vi "subBuildSpecAndReplaceLibrary.vi"(8 "error in (no error)":errorcluster, 9 "Spec and project refs":map{string, T2}(c390), 10 "FileInfo":T1, 11 "VI in":refnum<vi>) -> (0 "error out":errorcluster, 1 "Loose files":path[](array[path]), 2 "Result":string, 3 "Message":string)   [LabVIEW 2020, in "SolutionBuilder.lvlib" / "SolutionBuilder.lvclass"]
uses:
  SolutionBuilder.lvclass
  Private/SpecAndProject.ctl
  Private/FileInfo.ctl
  <vilib>/Utility/miscctls.llb/LVReplaceWithSaveOptionEnum.ctl
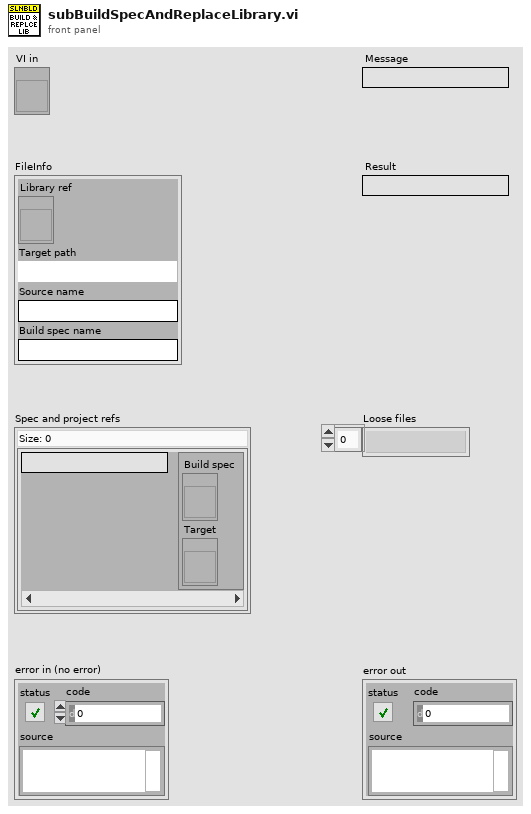
[diagram p1: front panel]
types:
  T1 = typedef "SolutionBuilder.lvlib/SolutionBuilder.lvclass/FileInfo.ctl" = cluster{"Library ref":refnum<vi>, "Target path":path, "Source name":string, "Build spec name":string}
  T2 = typedef "SolutionBuilder.lvlib/SolutionBuilder.lvclass/SpecAndProject.ctl" = cluster{"Build spec":refnum<vi>, "Target":refnum<vi>}
  T3 = typedef "LVReplaceWithSaveOptionEnum.ctl" = enum16{"Save All Without Prompts", "Save All With Prompts", "Do Not Save (Retain In Memory)"}
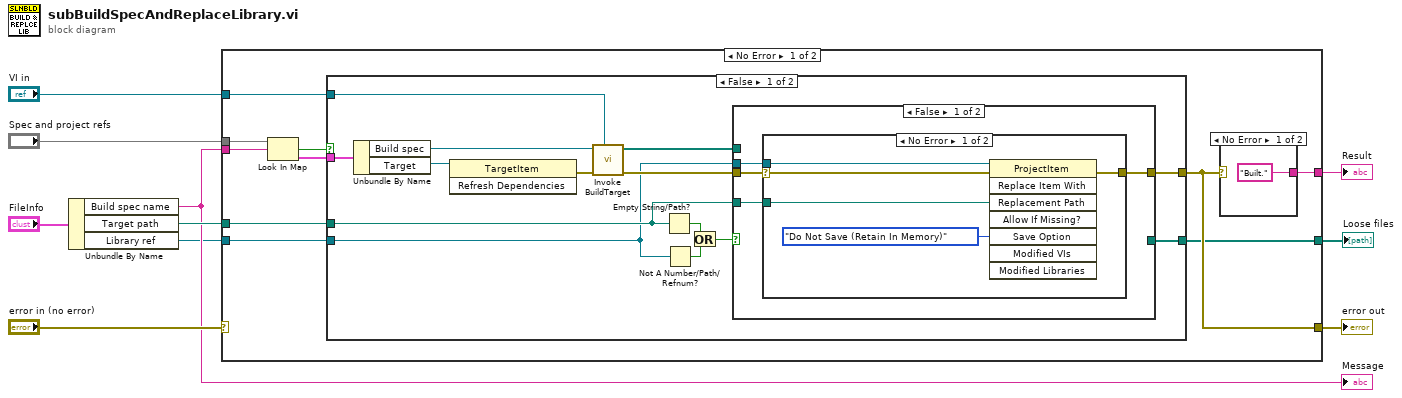
[diagram p0: block diagram]
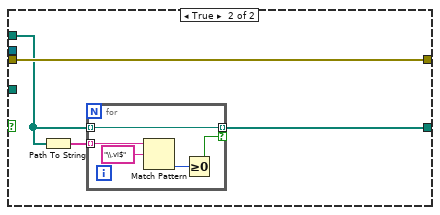
[diagram p3: hidden frame]
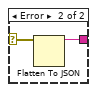
[diagram p5: hidden frame]
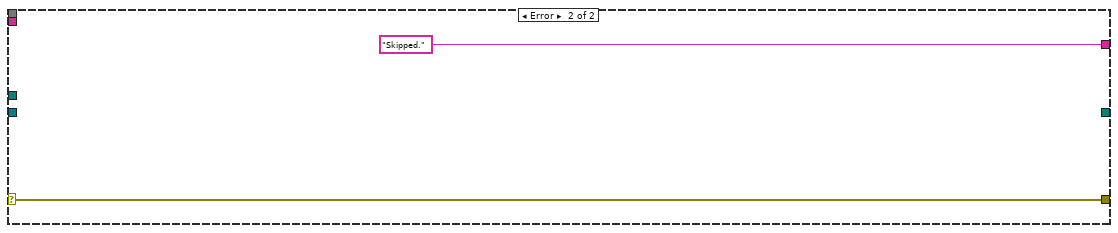
[diagram p6: hidden frame]
diagram:
  n1 = Unbundle By Name("FileInfo") -> ("Build spec name"=w3:string, "Target path"=w9:path, "Library ref"=w2:refnum<vi>)
  "Message" <- w3
  n2 = case shown="No Error" "error in (no error)" {
    selector: "error in (no error)" -> [_ w57]
    tunnel: "VI in" -> [w20 _]
    tunnel: w9 -> [w19 _]
    tunnel: w2 -> [w18 _]
    tunnel: "Spec and project refs" -> [w16 _]
    tunnel: w3 -> [w15 _]
    tunnel: [w13 "Skipped." ("JSON string")] -> w6
    tunnel: [w12 w57] -> w4
    tunnel: [w11 _] -> w1
    frame No Error {
      n3 = Look In Map(map=w16, key=w15) -> (key not found?=w14:bool, value=w17:T2)  [unwired: 1 in]
      n4 = case shown="False" w14 {
        tunnel: w20 -> [w34 _]
        tunnel: w19 -> [w31 _]
        tunnel: w18 -> [w30 _]
        tunnel: [w33 _] -> w12
        tunnel: w17 -> [w24 _]
        tunnel: [w25 _] -> w11
        frame False {
          n5 = Unbundle By Name(w24) -> ("Build spec"=w23:refnum<vi>, "Target"=w22:refnum<vi>)
          n6 = invoke class="TargetItem" method="Refresh Dependencies"(reference=w22) -> (error out=w21:errorcluster)  [unwired: 2 in, 2 out]
          n7 = call <vilib>:"Invoke BuildTarget.vi"("vi reference"=w34, "error in (no error)"=w21, "BuildItem ref"=w23) -> ("error out"=w32:errorcluster, "Generated files"=w26:path[])  [unwired: 7 in]
          n8 = Empty String/Path?(string/path=w31) -> (empty?=w29:bool)
          n9 = Not A Number/Path/Refnum?(number/path/refnum=w30) -> (NaN/Path/Refnum?=w28:bool)
          n10 = Or(x=w29, y=w28) -> (x .or. y?=w27:bool)
          n11 = case shown="False" w27 {
            tunnel: w31 -> [w38 _]
            tunnel: w30 -> [w37 _]
            tunnel: [w36 w48] -> w33
            tunnel: w32 -> [w35 w48]
            tunnel: w26 -> [_ w47]
            tunnel: [_ w45] -> w25
            frame False {
              n12 = case shown="No Error" w35 {
                selector: w35 -> [w43 w44]
                tunnel: [w39 w44] -> w36
                tunnel: w37 -> [w42 _]
                tunnel: w38 -> [w40 _]
                frame No Error {
                  n13 = invoke class="ProjectItem" method="Replace Item With"(reference=w42, error in=w43, "Replacement Path"=w40, "Save Option"=LVReplaceWithSaveOptionEnum."Do Not Save (Retain In Memory)") -> (error out=w39:errorcluster)  [unwired: 4 in, 7 out]
                }
                frame Error {
                }
              }
            }
            frame True {
              n14 = Path To String(path=w47) -> (string=w46:string[])
              n15 = for {
                tunnel: w47 -> [w50] mode=indexing
                tunnel: w46 -> [w53] mode=indexing
                tunnel: [w50] -> w45 mode=indexing if=w49
                n16 = Match Pattern(string=w53, regular expression="\\.vi$") -> (offset past match=w51:i32)  [unwired: 1 in, 3 out]
                n17 = Greater Or Equal To 0?(x=w51) -> (x >= 0?=w49:bool)
              }
            }
          }
        }
        frame True {
        }
      }
      n18 = case shown="No Error" w12 {
        selector: w12 -> [_ w56]
        tunnel: ["Built." ("f") w55] -> w13
        frame No Error {
        }
        frame Error {
          n19 = Flatten To JSON(anything=w56) -> (JSON string=w55:string)  [unwired: 2 in, 1 out]
        }
      }
    }
    frame Error {
    }
  }
  "Result" <- w6
  "error out" <- w4
  "Loose files" <- w1
